vi "Read Incoming Bytes.vi"(7 "mode (standard)":T1(ring), 8 "error in (no error)":errorcluster, 9 "timeout (1000 ms)":i32=1000, 10 "bytes to read (100)":i32=100, 11 "TCPConnection in":refnum<class "TCPConnection.lvclass">) -> (0 "error out":errorcluster, 1 "timed out":bool, 2 "Bytes":u8[](array[numeric]) format="%08b", 3 "TCPConnection out":refnum<class "TCPConnection.lvclass">)   [LabVIEW 2013, in "MQTT Server.lvlib" / "TCPConnection.lvclass"]
uses:
  TCPConnection.lvclass
  TCPConnection.lvclass/TCPConnection.ctl
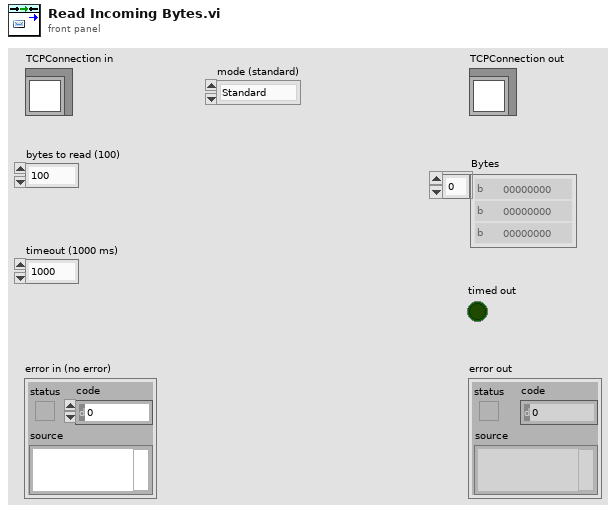
[diagram p1: front panel]
types:
  T1 = enum16{"Standard", "Buffered", "CRLF", "Immediate"}
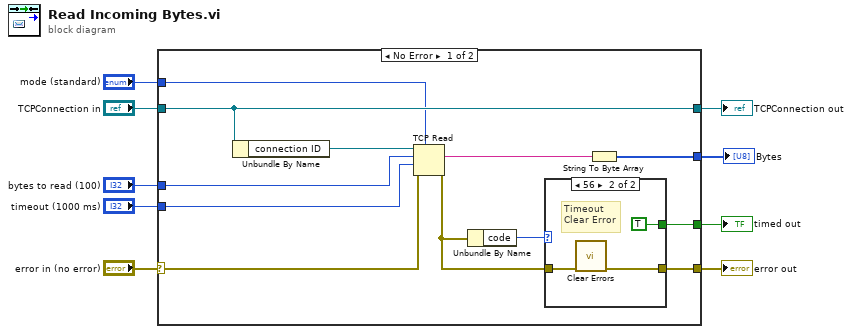
[diagram p0: block diagram]
diagram:
  n1 = case shown="No Error" "error in (no error)" {
    selector: "error in (no error)" -> [w19 w27]
    tunnel: [w15 w27] -> w8
    tunnel: [w21 w26] -> w6
    tunnel: "TCPConnection in" -> [w21 w26]
    tunnel: [w17 _] -> w5
    tunnel: "bytes to read (100)" -> [w13 _]
    tunnel: "timeout (1000 ms)" -> [w12 _]
    tunnel: [w11 _] -> w2
    tunnel: "mode (standard)" -> [w10 _]
    frame No Error {
      n2 = Unbundle By Name(w21) -> ("connection ID"=w20:refnum<k5>)
      n3 = TCP Read(connection ID=w20, bytes to read=w13, error in (no error)=w19, 7:w10, 9:w12) -> (data out=w18:string, error out=w14:errorcluster)  [unwired: 1 out]
      n4 = Unbundle By Name(w14) -> ("code"=w16:i32)
      n5 = case shown="56" w16 {
        tunnel: [w22 w25] -> w15
        tunnel: w14 -> [w22 w24]
        tunnel: [_ TRUE] -> w11
        frame Default {
        }
        frame 56 {
          # "Timeout\nClear Error"
          n6 = call <vilib>:"Clear Errors.vi"("error in (no error)"=w24) -> ("error out"=w25:errorcluster)  [unwired: 6 in]
        }
      }
      n7 = String To Byte Array(string=w18) -> (unsigned byte array=w17:u8[])
    }
    frame Error {
    }
  }
  "error out" <- w8
  "TCPConnection out" <- w6
  "Bytes" <- w5
  "timed out" <- w2
